vi "GB_Serial Test.vi"(8 "error in (no error)":errorcluster) -> (0 "error out":errorcluster, 1 "Pass/Fail":bool, 2 "VISA resource OUT":refnum<visa-resource-name>, 3 "Actual Result":string, 7 "Expected Result":string)   [LabVIEW 2022 SP3]
uses:
  <vilib>/Instr/_visa.llb/VISA Flush IO Buffer Mask.ctl
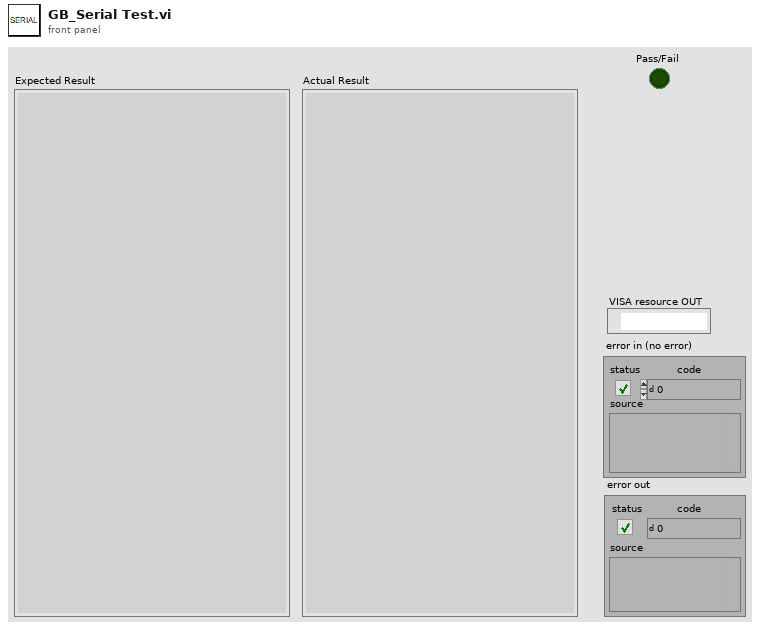
[diagram p1: front panel]
types:
  T1 = typedef "VISA Flush IO Buffer Mask.ctl" = u16
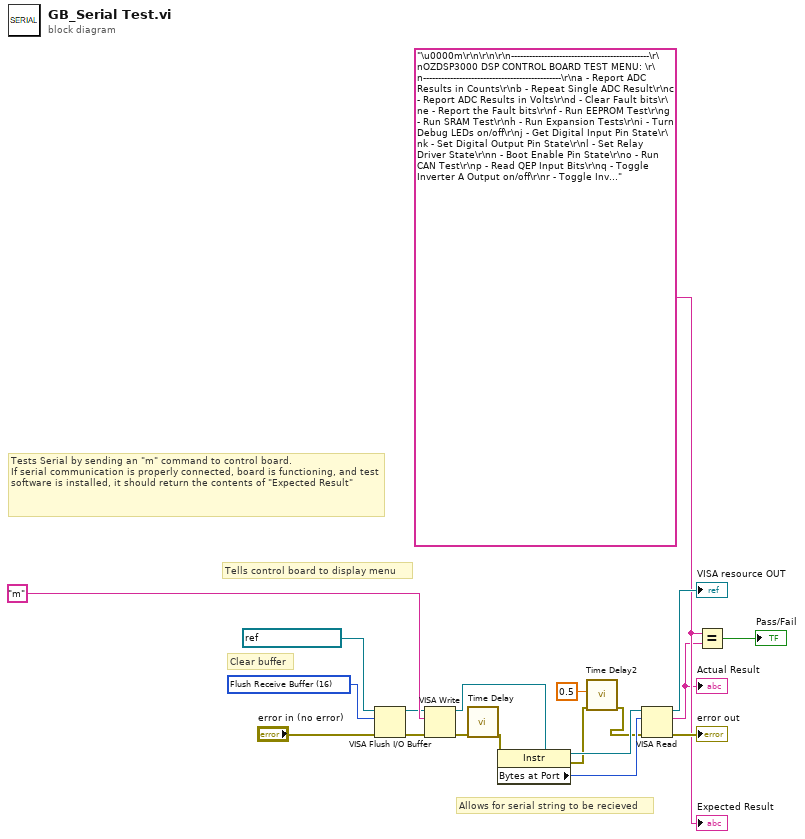
[diagram p0: block diagram]
diagram:
  w7 = "\u0000m\r\n\r\n\r\n----------------------------------------------\r\nOZDSP3000 DSP CONTROL BOARD TEST MENU: \r\n----------------------------------------------\r\na - Report ADC Results in Counts\r\nb - Repeat Single ADC Result\r\nc - Report ADC Results in Volts\r\nd - Clear Fault bits\r\ne - Report the Fault bits\r\nf - Run EEPROM Test\r\ng - Run SRAM Test\r\nh - Run Expansion Tests\r\ni - Turn Debug LEDs on/off\r\nj - Get Digital Input Pin State\r\nk - Set Digital Output Pin State\r\nl - Set Relay Driver State\r\nn - Boot Enable Pin State\r\no - Run CAN Test\r\np - Read QEP Input Bits\r\nq - Toggle Inverter A Output on/off\r\nr - Toggle Inverter B Output on/off\r\ns - Toggle Half Bridge Output on/off\r\nt - Set PWM leg duty cycle\r\nu - Real Time Clock\r\nv - Watchdog Control\r\nw - Test Interrupt Lines\r\nx - Read HALLs\r\ny - Test FPGA Read/Write\r\nz - Report Software/FPGA Revs\r\nm - Display this menu\r\n> \u0000"
  w16 = T1 16 items=["Flush Receive Buffer"=16, "Write Transmit Buffer to Device"=32, "Flush Receive Buffer (No I/O)"=64, "Flush Transmit Buffer"=128] ("Mask")
  # "Tests Serial by sending an \"m\" command to control board.\nIf serial communication is properly connected, board is functioning, and test software is installed, it should return the contents of \"Expected Result\""
  # "Clear buffer"
  # "Allows for serial string to be recieved"
  # "Tells control board to display menu"
  n1 = VISA Flush I/O Buffer(VISA resource name=refnum<visa-resource-name> "ControlBoard", mask (16)=w16, error in (no error)="error in (no error)") -> (VISA resource name out=w14:refnum<visa-resource-name>, error out=w13:errorcluster)
  n2 = VISA Write(VISA resource name=w14, write buffer="m", error in (no error)=w13) -> (VISA resource name out=w11:refnum<visa-resource-name>, error out=w15:errorcluster)  [unwired: 1 out]
  n3 = call "Time Delay"("error in (no error)"=w15) -> ("error out"=w12:errorcluster)  [unwired: 10 in]
  n4 = property class="Instr"(reference=w11, error in=w12) -> (reference out=w18:refnum<visa-resource-name>, error out=w3:errorcluster, "Bytes at Port"=w17:u32)
  n5 = call "Time Delay2"("error in (no error)"=w3, "Delay Time (s)"=0.5) -> ("error out"=w2:errorcluster)  [unwired: 9 in]
  n6 = VISA Read(VISA resource name=w18, byte count=w17, error in (no error)=w2) -> (VISA resource name out=→"VISA resource OUT":refnum<visa-resource-name>, read buffer=w6:string, error out=→"error out":errorcluster)  [unwired: 1 out]
  "Actual Result" <- w6
  n7 = Equal?(x=w7, y=w6) -> (x = y?=→"Pass/Fail":bool)
  "Expected Result" <- w7
